vi "Disabled.vi"(7 "Robot Mode":T2, 10 "Match Info":T1={"Autonomous Elapsed Seconds"=0.0, "TeleOp Elapsed Seconds"=0.0, "Disabled Elapsed Seconds"=0.0, "Visited Autonomous"=FALSE, "Visited TeleOp"=FALSE, "Visited Disabled"=FALSE, "Autonomous Settings"={"Autonomous Style"=enum."Independent", "VI Refnum"=refnum}}, 11 "Call Context":T3) -> ()   [LabVIEW 2012]
doc: "This VI is called each time a disabled packet is received from the DS. It is often used to prepare for the next robot mode, to calibrate sensors, etc."
uses:
  <vilib>/Rock Robotics/WPI/DriverStation/WPI_DriverStationDerivedRobotMode.ctl
  <vilib>/Rock Robotics/WPI/DriverStation/WPI_DriverStationRobotMode2.ctl
  <vilib>/Rock Robotics/WPI/DriverStation/WPI_DriverStationMatch Info.ctl
  Robot Global Data.vi
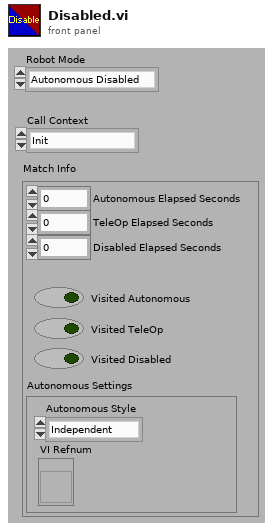
[diagram p1: front panel]
types:
  T1 = typedef "WPI_DriverStationMatch Info.ctl" = cluster{"Autonomous Elapsed Seconds":dbl, "TeleOp Elapsed Seconds":dbl, "Disabled Elapsed Seconds":dbl, "Visited Autonomous":bool, "Visited TeleOp":bool, "Visited Disabled":bool, "Autonomous Settings":cluster{"Autonomous Style":enum16{"Iterative", "Independent"}, "VI Refnum":refnum<vi>}}
  T2 = typedef "WPI_DriverStationRobotMode2.ctl" = enum16{"Autonomous Disabled", "Autonomous Enabled", "Teleop Disabled", "Teleop Enabled", "Timeout", "Finish", "Test Disabled", "Test Enabled"}
  T3 = typedef "WPI_DriverStationDerivedRobotMode.ctl" = enum16{"Init", "Execute", "Stop"}
  T4 = typedef "WPI_MotorControlDeviceRef.ctl" = cluster{"DeviceStatus":errorcluster, "Type":enum16{"PWM", "CAN"}, "PWM":cluster{"Digital Module":T5, "PWM Channel":T6, "DeadBand":T7}, "CAN":cluster{"Device Number":u8, "Control Mode":T8, "Semaphore":T9, "Max Vout":dbl}, "Invert":bool, "TransformRef":T10, "InvTransformRef":T10}
  T5 = typedef "FPGA_TypedefDigitalModule.ctl" = enum16{"Digital Module 1", "Digital Module 2"}
  T6 = typedef "FPGA_DIOPWMChannel.ctl" = enum8{"PWM 1", "PWM 2", "PWM 3", "PWM 4", "PWM 5", "PWM 6", "PWM 7", "PWM 8", "PWM 9", "PWM 10", "Invalid"}
  T7 = typedef "WPI_PWMDeadband.ctl" = cluster{"Name":string, "maxPositivePwm":i32, "minPositivePwm":i32, "centerPwm":i32, "maxNegativePwm":i32, "minNegativePwm":i32, "angularRange":u16}
  T8 = typedef "WPI_CANJaguar_ControlMode.ctl" = enum8{"Percent VBus", "Current", "Speed", "Position", "Voltage"}
  T9 = typedef "Semaphore RefNum" = refnum<k1>
  T10 = typedef "WPI_PWMTransform_ConPane.ctl" = refnum<vi>
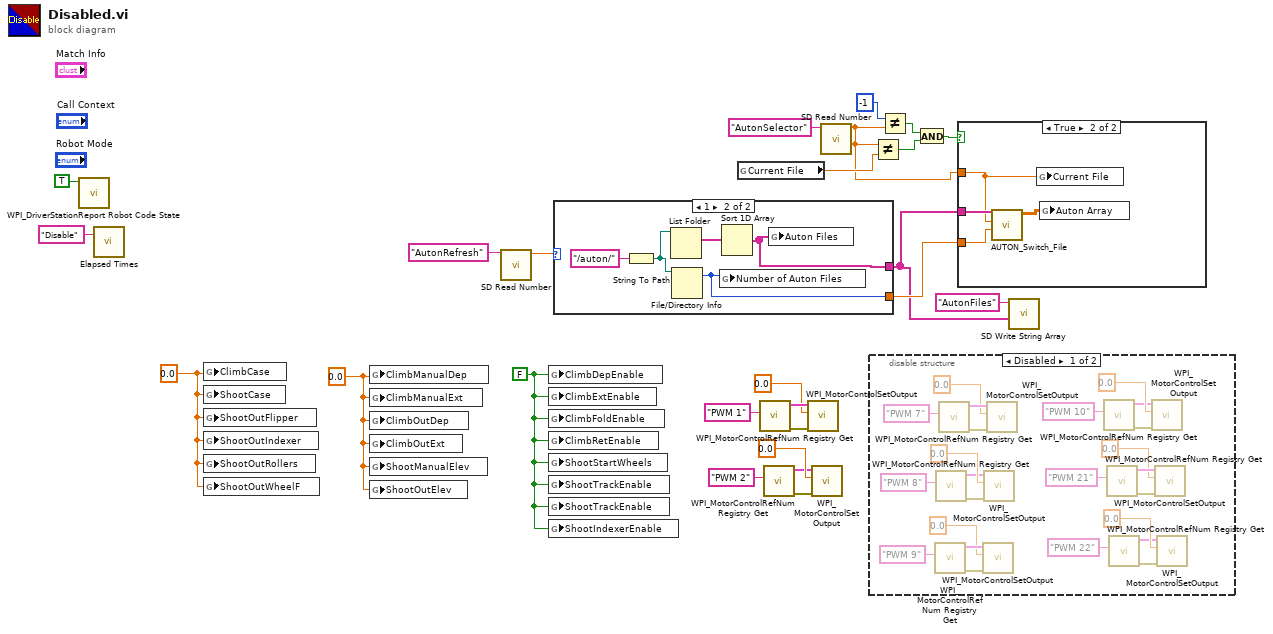
[diagram p0: block diagram]
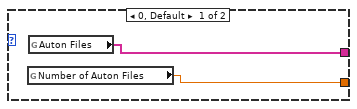
[diagram p4: hidden frame]
diagram:
  w1 = FALSE ("ClimbDepEnable")
  w2 = 0.0 ("ClimbCase")
  w3 = 0.0 ("ClimbCase")
  n1 = call <vilib>:"WPI_DriverStationReport Robot Code State.vi"("Disabled"=TRUE ("Autonomous")) -> ()  [unwired: 10 in, 1 out]
  n2 = call "Elapsed Times.vi"("Call Name"="Disable") -> ()  [unwired: 2 in, 1 out]
  n3 = global write "Robot Global Data.vi" "ClimbCase"(w3) -> ()
  n4 = global write "Robot Global Data.vi" "ShootCase"(w3) -> ()
  n5 = global write "Robot Global Data.vi" "ShootOutFlipper"(w3) -> ()
  n6 = global write "Robot Global Data.vi" "ShootOutIndexer"(w3) -> ()
  n7 = global write "Robot Global Data.vi" "ShootOutRollers"(w3) -> ()
  n8 = global write "Robot Global Data.vi" "ShootOutWheelF"(w3) -> ()
  n9 = global write "Robot Global Data.vi" "ClimbManualDep"(w2) -> ()
  n10 = global write "Robot Global Data.vi" "ClimbManualExt"(w2) -> ()
  n11 = global write "Robot Global Data.vi" "ClimbOutDep"(w2) -> ()
  n12 = global write "Robot Global Data.vi" "ClimbOutExt"(w2) -> ()
  n13 = global write "Robot Global Data.vi" "ShootManualElev"(w2) -> ()
  n14 = global write "Robot Global Data.vi" "ShootOutElev"(w2) -> ()
  n15 = call <vilib>:"SD Read Number.vi"("Name"="AutonRefresh") -> ("Numeric"=w5:dbl)  [unwired: 8 in, 2 out]
  n16 = global write "Robot Global Data.vi" "ClimbDepEnable"(w1) -> ()
  n17 = global write "Robot Global Data.vi" "ClimbExtEnable"(w1) -> ()
  n18 = global write "Robot Global Data.vi" "ClimbFoldEnable"(w1) -> ()
  n19 = global write "Robot Global Data.vi" "ClimbRetEnable"(w1) -> ()
  n20 = global write "Robot Global Data.vi" "ShootStartWheels"(w1) -> ()
  n21 = global write "Robot Global Data.vi" "ShootTrackEnable"(w1) -> ()
  n22 = global write "Robot Global Data.vi" "ShootTrackEnable"(w1) -> ()
  n23 = global write "Robot Global Data.vi" "ShootIndexerEnable"(w1) -> ()
  n24 = case shown="1" w5 {
    tunnel: [w26 w29] -> w15
    tunnel: [w27 w28] -> w10
    frame 0, Default {
      n25 = global read "Robot Global Data.vi" "Number of Auton Files"() -> (w26:dbl)
      n26 = global read "Robot Global Data.vi" "Auton Files"() -> (w27:string[])
    }
    frame 1 {
      n27 = String To Path(string="/auton/") -> (path=w31:path)
      n28 = List Folder(path=w31) -> (filenames=w30:string[])  [unwired: 3 in, 3 out]
      n29 = File/Directory Info(path=w31) -> (size=w29:i64)  [unwired: 1 in, 6 out]
      n30 = global write "Robot Global Data.vi" "Number of Auton Files"(w29) -> ()
      n31 = Sort 1D Array(array=w30) -> (sorted array=w28:string[])
      n32 = global write "Robot Global Data.vi" "Auton Files"(w28) -> ()
    }
  }
  n33 = global read "Robot Global Data.vi" "Current File"() -> (w13:dbl)
  n34 = call <vilib>:"WPI_MotorControlRefNum Registry Get.vi"("refnum name"="PWM 1") -> ("error out"=w23:errorcluster, "MotorControlDevRef"=w22:T4)  [unwired: 9 in]
  n35 = call <vilib>:"WPI_MotorControlRefNum Registry Get.vi"("refnum name"="PWM 2") -> ("error out"=w16:errorcluster, "MotorControlDevRef"=w17:T4)  [unwired: 9 in]
  n36 = call <vilib>:"WPI_MotorControlSetOutput.vi"("error in (no error)"=w23, "Output"=0.0, "MotorControlDevRef"=w22) -> ()  [unwired: 6 in, 3 out]
  n37 = call <vilib>:"WPI_MotorControlSetOutput.vi"("error in (no error)"=w16, "Output"=0.0, "MotorControlDevRef"=w17) -> ()  [unwired: 6 in, 3 out]
  n38 = call <vilib>:"SD Read Number.vi"("Name"="AutonSelector") -> ("Numeric"=w6:dbl)  [unwired: 8 in, 2 out]
  n39 = disable-structure shown="Disabled" {
    frame Disabled {
      n40 = call <vilib>:"WPI_MotorControlRefNum Registry Get.vi"("refnum name"="PWM 9") -> ("error out"=w48:errorcluster, "MotorControlDevRef"=w47:T4)  [unwired: 9 in]
      n41 = call <vilib>:"WPI_MotorControlRefNum Registry Get.vi"("refnum name"="PWM 8") -> ("error out"=w49:errorcluster, "MotorControlDevRef"=w50:T4)  [unwired: 9 in]
      n42 = call <vilib>:"WPI_MotorControlRefNum Registry Get.vi"("refnum name"="PWM 7") -> ("error out"=w56:errorcluster, "MotorControlDevRef"=w55:T4)  [unwired: 9 in]
      n43 = call <vilib>:"WPI_MotorControlSetOutput.vi"("error in (no error)"=w48, "Output"=0.0, "MotorControlDevRef"=w47) -> ()  [unwired: 6 in, 3 out]
      n44 = call <vilib>:"WPI_MotorControlSetOutput.vi"("error in (no error)"=w49, "Output"=0.0, "MotorControlDevRef"=w50) -> ()  [unwired: 6 in, 3 out]
      n45 = call <vilib>:"WPI_MotorControlSetOutput.vi"("error in (no error)"=w56, "Output"=0.0, "MotorControlDevRef"=w55) -> ()  [unwired: 6 in, 3 out]
      n46 = call <vilib>:"WPI_MotorControlRefNum Registry Get.vi"("refnum name"="PWM 10") -> ("error out"=w41:errorcluster, "MotorControlDevRef"=w42:T4)  [unwired: 9 in]
      n47 = call <vilib>:"WPI_MotorControlRefNum Registry Get.vi"("refnum name"="PWM 21") -> ("error out"=w40:errorcluster, "MotorControlDevRef"=w39:T4)  [unwired: 9 in]
      n48 = call <vilib>:"WPI_MotorControlRefNum Registry Get.vi"("refnum name"="PWM 22") -> ("error out"=w33:errorcluster, "MotorControlDevRef"=w34:T4)  [unwired: 9 in]
      n49 = call <vilib>:"WPI_MotorControlSetOutput.vi"("error in (no error)"=w41, "Output"=0.0, "MotorControlDevRef"=w42) -> ()  [unwired: 6 in, 3 out]
      n50 = call <vilib>:"WPI_MotorControlSetOutput.vi"("error in (no error)"=w40, "Output"=0.0, "MotorControlDevRef"=w39) -> ()  [unwired: 6 in, 3 out]
      n51 = call <vilib>:"WPI_MotorControlSetOutput.vi"("error in (no error)"=w33, "Output"=0.0, "MotorControlDevRef"=w34) -> ()  [unwired: 6 in, 3 out]
    }
    frame Enabled {
    }
  }
  n52 = Not Equal?(x=w6, y=w13) -> (x != y?=w11:bool)
  n53 = Not Equal?(x=-1, y=w6) -> (x != y?=w12:bool)
  n54 = And(x=w12, y=w11) -> (x .and. y?=w8:bool)
  n55 = case shown="True" w8 {
    tunnel: w10 -> [_ w60]
    tunnel: w15 -> [_ w59]
    tunnel: w6 -> [_ w57]
    frame False {
    }
    frame True {
      n56 = call "AUTON_Switch_File.vi"("Number of Auton Files"=w59, "Auton File"=w57, "Auton Files"=w60) -> ("Auton Array"=w58:dbl[][])  [unwired: 7 in, 1 out]
      n57 = global write "Robot Global Data.vi" "Current File"(w57) -> ()
      n58 = global write "Robot Global Data.vi" "Auton Array"(w58) -> ()
    }
  }
  n59 = call <vilib>:"SD Write String Array.vi"("String Array"=w10, "Name"="AutonFiles") -> ()  [unwired: 8 in, 2 out]
